vi "Configure Reference Wavefrom.vi"   [LabVIEW 2015, in "Agilent 2000 3000 X-Series.lvlib"]
doc: "Configures reference waveform.\n\n<B>Note(s):</B>\nThis VI has been obsoleted from the driver and is included for compatibility with existing applications. New applications should use the Configure Referehce Waveform VI."
uses:
  <instrlib>/Agilent 2000 3000 X-Series/Agilent 2000 3000 X-Series.lvlib
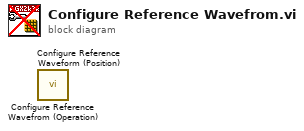
[diagram p0: block diagram]
diagram:
  n1 = call <instrlib>:"Configure Reference Wavefrom (Operation).vi"() -> ()  [unwired: 10 in, 2 out]
  n2 = call <instrlib>:"Configure Reference Waveform (Position).vi"() -> ()  [unwired: 10 in, 2 out]
